vi "DIFF_DRIVE_GET_SPEED_DEMAND.vi"() -> (0 "Drv Rotation Orentation Dmd":dbl, 1 "Drv Angular Vel Dmd":dbl, 2 "Drv Y Vel Dmd":dbl, 3 "Drv X Vel Dmd":dbl)   [LabVIEW 2023]
uses:
  DIFF_DRIVE_GLOBALS.vi
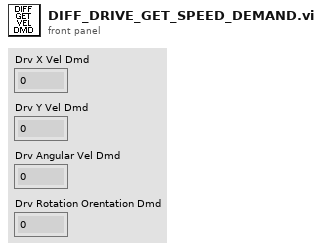
[diagram p1: front panel]
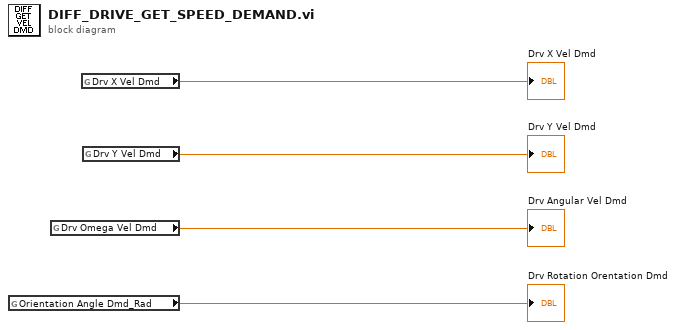
[diagram p0: block diagram]
diagram:
  n1 = global read "DIFF_DRIVE_GLOBALS.vi" "Orientation Angle Dmd_Rad"() -> (→"Drv Rotation Orentation Dmd":dbl)
  n2 = global read "DIFF_DRIVE_GLOBALS.vi" "Drv Omega Vel Dmd"() -> (→"Drv Angular Vel Dmd":dbl)
  n3 = global read "DIFF_DRIVE_GLOBALS.vi" "Drv X Vel Dmd"() -> (→"Drv X Vel Dmd":dbl)
  n4 = global read "DIFF_DRIVE_GLOBALS.vi" "Drv Y Vel Dmd"() -> (→"Drv Y Vel Dmd":dbl)
